vi "NIMS_NS_iir_grpdelay.vi"(5 "Function name":string, 6 "Line number":i32, 7 "Number of outputs requested":i32, 8 "error in (no error)":errorcluster, 11 "[A]":variant[](array[variant])) -> (0 "error out":errorcluster, 3 "[funct(A)]":variant[](array[variant]))   [LabVIEW 2017]
uses:
  <vilib>/imath/engines/lvmath/Functions/Error Handling/error.ctl
  <instcachedir>/0/NIMS_RunTimeType_From StrictType (excl LVString)_1019F277F0A747EDBCA0F6C52CA54500.lvgen/NIMS_RunTimeType_From StrictType (excl LVString)_1019F277F0A747EDBCA0F6C52CA54500_000.vi
  <instcachedir>/0/NIMS_Get Scalar_w Error_1987D997E87247DDAC16EA23A5E9E4FC.lvgen/NIMS_Get Scalar_w Error_1987D997E87247DDAC16EA23A5E9E4FC_000.vi
  <instcachedir>/0/NIMS_Complex To Real_BE01396FDE034E8E94CEBBA1E368668D.lvgen/NIMS_Complex To Real_BE01396FDE034E8E94CEBBA1E368668D_000.vi
  <instcachedir>/0/NIMS_Get Any Vector_w Error - Matrix_9FDB8FBE264C42EDBC8FF9BA66C3EF33.lvgen/NIMS_Get Any Vector_w Error - Matrix_9FDB8FBE264C42EDBC8FF9BA66C3EF33_001.vi
  <instcachedir>/0/NIMS_Get Scalar_w Error_1987D997E87247DDAC16EA23A5E9E4FC.lvgen/NIMS_Get Scalar_w Error_1987D997E87247DDAC16EA23A5E9E4FC_003.vi
  <instcachedir>/0/NIMS_RunTimeType_To Numeric_1CBDAFC4EFAD4045A1DE52278D16738D.lvgen/NIMS_RunTimeType_To Numeric_1CBDAFC4EFAD4045A1DE52278D16738D_000.vi
  <vilib>/addons/Digital Filter Design/NI_DigFilter_MathScript.lvlib
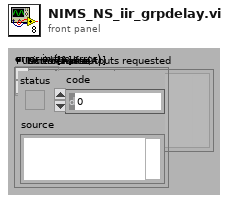
[diagram p1: front panel]
types:
  T1 = typedef "error.ctl" = enum16{"No Error", "Problem", "Input type must not be void", "Incorrect number of parameters", "Function not defined for non-numeric types", "An output variable of the user-defined function is undefined", "Function only defined for character arrays", "Function not defined for boolean, character, or single precision", "Function not defined for complex types", "Not a valid operation", "Inputs must be scalar", "Input matrices are not the same size", "Function only available on RT", "Input matrices must be nonnegative integers of the same type", "Arguments must be non-negative integers less than bitmax", "Number to complement must be less than 2^N", "Bit to get is outside range", "Bit to set is outside range", "Input must be real type ", "At least one parameter must be scalar", "Unable to display plug-in data on RT", "Function not defined for higher dimensional matrices", "Invalid attributes", "Wrong Type of Input Arguments", "Wrong Argument Option", "Invalid file identifier", "Indices must be real positive integers", "The variable is not a matrix data type.", "Number of elements must be the same for indices and values", "You cannot replace elements of a matrix with non-matrix data types.", "Cannot resize a 2D matrix with a linear index", "Unknown variable or symbol", "Indices out of range", "Empty matrix deletion can not be used with two indices", "Number of rows and columns must be the same for indices and values.", "Complex cannot be converted to Boolean", "Char cannot be converted to Boolean", "int64 cannot be converted to Boolean", "uint64 cannot be converted to Boolean", "You cannot convert a Boolean to a character.", "Incompatible input size in 3D surface function", "All rows must have the same number of columns", "Incompatible types", "Invalid matrix dimensions", "Dimension must be 1 or 2", "Base must be an integer between 2 and 36", "Invalid input", "Square matrix required", "Function 'timerstart' must be called before 'timerstop'", "Arguments must be positive real", "Step must not be zero", "Wrong number of input arguments", "Wrong number of output arguments", "Too many index arguments", "Input scalar must be >= 0", "Input scalar must be positive", "Input scalar must not be 0", "Input scalar must be in range [0,1]", "Can't use conditionally defined variable that's undefined", "Input must be a vector", "RT Exec Trace Toolkit not licensed", "Empty vector error", "All elements must be in domain [-1,1]", "All real elements of input vector must be >= 0", "All elements of input vector must be positive", "Values of input vectors are not compatible", "DAQmx not installed", "Input vector must be an increasing vector", "Dereferenced field does not exist within the struct", "A vector or matrix of structures must be indexed before it can be dereferenced", "Lenths of two input vectors are not compatible", "Invalid fieldname", "Empty matrix error", "Cannot use '.' on a type other than Struct", "Unused074", "Data type of the struct's field name is invalid", "Using . to dereference data that is not a struct", "Input struct contains invalid type ", "Size of input matrix is incompatible with input size", "Invalid format specifier", "Could not find field within struct", "Bad permutation array", "Mismatched fieldnames", "ode: User Function could not be opened", "ode: User Function signature does not meet ode requirements", "Unused085", "RunTime: MathScript could not be compiled", "Unknown function", "Only scalars and strings supported", "ode: User Function signature has incorrect number of inputs", "ode:User Function signature has incorrect number of outputs", "Range is too large", "End used without variable", "Function not available (RTE)", "Custom user error", "Arguments must be integers less than bitmax", "Shared library not found", "Header file not found", "Shared library already loaded", "Shared library not loaded", "Shared library function not found", "Shared library string return problem", "Problem calling shared library function", "Problem loading shared library from OS", "Problem parsing shared library header file", "Shared library incompatible types", "Shared library unsupported return type", "Shared library function not exported", "Shared library unsupported input type", "Problem unloading shared library from OS", "Function only available from UI", "Function specified in argument is missing", "An internal error has occurred", "Invalid object", "Invalid property", "Read-only property", "A break command has occurred", "A continue command has occurred", "A return command has occurred", "ode: times parameter invalid", "Function specified in argument has incorrect signature", "Function not found in file", "Reserved keyword cannot be defined as variable", "Reserved keyword cannot be defined as a function or script", "Arguments must be string literals", "Function not supported on this platform", "All columns must have the same number of rows", "Function ignored in RTE warning", "Cannot use : as a parameter that is not a variable", "Output can't be coerced to requested type", "Function not supported on current target", "Variable dependent on an unwired function input", "Unused132", "Unused133", "Unused134", "Unused135", "Unused136", "Unused137", "Unused138", "Unused139", "Global/Persistent must only take constants as arguments.", "Varargin must be last input in the function definition.", "Varargout must be last output in the function definition.", "Invalid output type. Cannot output a cell array of any type other than string.", "Invalid output type. Type is a dynamic struct.", "Invalid output type. Type is a struct that has a field whose type is not known until run-time", "Invalid output type. Type is a struct that has a field which is a plot object.", "MathScript parser DLL missing", "MathScript requires LabVIEW Full", "MathScript license is invalid or missing", "Varargout not supported except in assignments."}
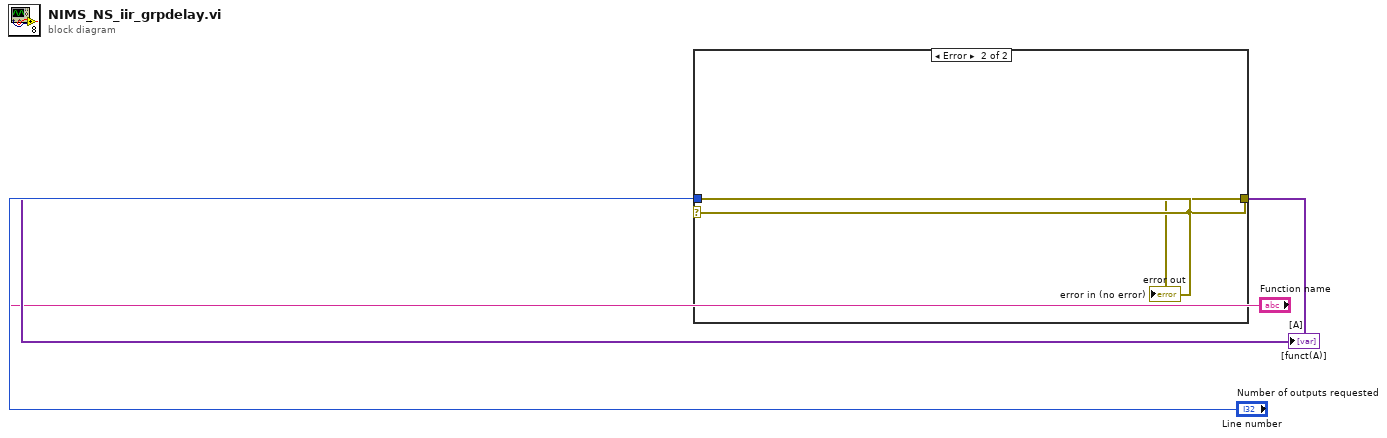
[diagram p0: block diagram]
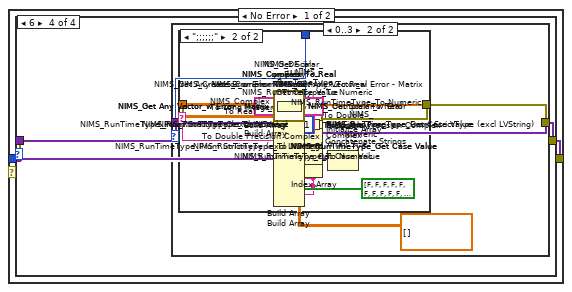
[diagram p2: hidden frame]
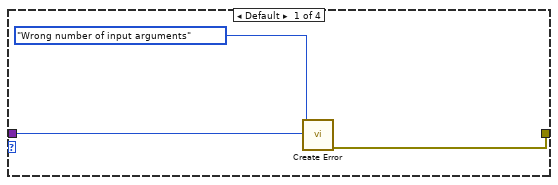
[diagram p3: hidden frame]
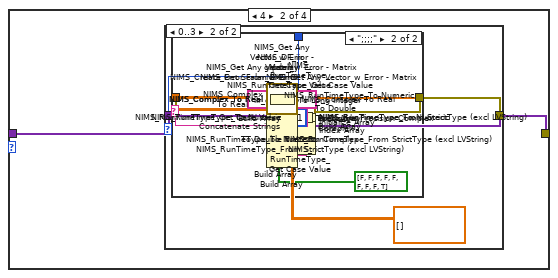
[diagram p4: hidden frame]
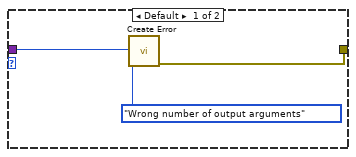
[diagram p5: hidden frame]
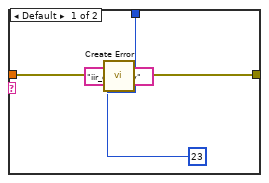
[diagram p6: hidden frame]
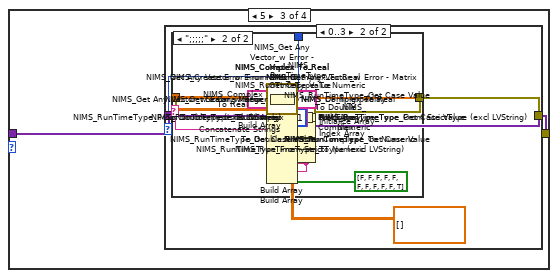
[diagram p7: hidden frame]
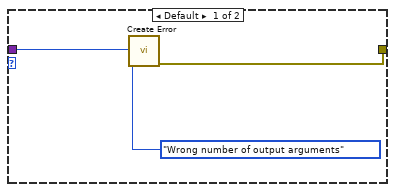
[diagram p8: hidden frame]
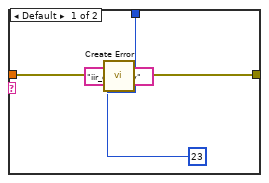
[diagram p9: hidden frame]
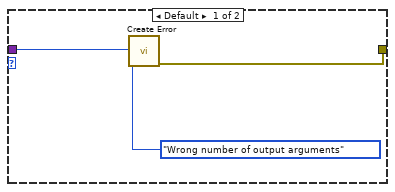
[diagram p10: hidden frame]
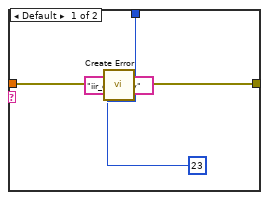
[diagram p11: hidden frame]
diagram:
  n1 = case shown="Error" "error in (no error)" {
    selector: "error in (no error)" -> [_ w312]
    tunnel: [w15 _] -> w4
    tunnel: [w14 w312] -> w3
    tunnel: "error in (no error)" -> [w13 _]
    tunnel: "Number of outputs requested" -> [w12 _]
    tunnel: "[A]" -> [w11 _]
    tunnel: "Function name" -> [w10 _]
    tunnel: "Line number" -> [w9 _]
    frame No Error {
      n2 = Array Size(array=w11) -> (size(s)=w8:i32)
      n3 = case shown="6" w8 {
        tunnel: [_ w27 w115 w212] -> w15
        tunnel: w10 -> [w19 w24 w112 w209]
        tunnel: w9 -> [w20 w25 w113 w210]
        tunnel: w13 -> [w17 w23 w111 w208]
        tunnel: [w16 w22 w110 w207] -> w14
        tunnel: w12 -> [_ w21 w109 w206]
        tunnel: w11 -> [_ w26 w114 w211]
        frame Default {
          n4 = call <vilib>:"Create Error.vi"("Function name"=w19, "error in (no error)"=w17, "Error Enum"=error."Wrong number of input arguments", "Line number"=w20) -> ("error out"=w16:errorcluster)  [unwired: 6 in, 1 out]
        }
        frame 4 {
          n5 = case shown="0..3" w21 {
            tunnel: [_ w33] -> w27
            tunnel: w24 -> [w31 _]
            tunnel: w25 -> [w32 w69]
            tunnel: w23 -> [w29 w67]
            tunnel: [w28 w50] -> w22
            tunnel: w26 -> [_ w70]
            frame Default {
              n6 = call <vilib>:"Create Error.vi"("Function name"=w31, "error in (no error)"=w29, "Error Enum"=error."Wrong number of output arguments", "Line number"=w32) -> ("error out"=w28:errorcluster)  [unwired: 6 in, 1 out]
            }
            frame 0..3 {
              w40 = 1
              n7 = Index Array(array=w70) -> (element #1=w66:variant, element #2=w62:variant, element #3=w58:variant, element #4=w54:variant)  [unwired: 4 in]
              n8 = call <vilib>:"NIMS_RunTimeType_Get Case Value.vi"("Data In"=w54) -> ("Case Value"=w51:string)  [unwired: 9 in, 1 out]
              n9 = call-generic <vilib>:"NIMS_RunTimeType_To Numeric.vi"("DataType"=cdb[][] [], "Variant"=w54) -> ("data"=w52:cdb[][])  [unwired: 1 in]
              n10 = call <vilib>:"NIMS_RunTimeType_Get Case Value.vi"("Data In"=w58) -> ("Case Value"=w55:string)  [unwired: 9 in, 1 out]
              n11 = call-generic <vilib>:"NIMS_RunTimeType_To Numeric.vi"("DataType"=cdb[][] [], "Variant"=w58) -> ("data"=w56:cdb[][])  [unwired: 1 in]
              n12 = call <vilib>:"NIMS_RunTimeType_Get Case Value.vi"("Data In"=w62) -> ("Case Value"=w59:string)  [unwired: 9 in, 1 out]
              n13 = call-generic <vilib>:"NIMS_RunTimeType_To Numeric.vi"("DataType"=cdb[][] [], "Variant"=w62) -> ("data"=w60:cdb[][])  [unwired: 1 in]
              n14 = call <vilib>:"NIMS_RunTimeType_Get Case Value.vi"("Data In"=w66) -> ("Case Value"=w63:string)  [unwired: 9 in, 1 out]
              n15 = call-generic <vilib>:"NIMS_RunTimeType_To Numeric.vi"("DataType"=cdb[][] [], "Variant"=w66) -> ("data"=w64:cdb[][])  [unwired: 1 in]
              n16 = Concatenate Strings(w63, w59, w55, w51) -> (w68:string)
              n17 = case shown="\";;;;\"" w68 {
                tunnel: w67 -> [w72 w83]
                tunnel: [_ w78] -> w49
                tunnel: [_ w77] -> w45
                tunnel: [_ w76] -> w41
                tunnel: [w71 w79] -> w50
                tunnel: w64 -> [_ w107]
                tunnel: w60 -> [_ w103]
                tunnel: w56 -> [_ w100]
                tunnel: w52 -> [_ w97]
                tunnel: w69 -> [w75 w86]
                frame Default {
                  n18 = call <vilib>:"Create Error.vi"("Function name"="iir_grpdelay", "error in (no error)"=w72, "Error Enum"=23, "Line number"=w75) -> ("error out"=w71:errorcluster)  [unwired: 6 in, 1 out]
                }
                frame ";;;;" {
                  w81 = "iir_grpdelay"
                  n19 = call-generic <vilib>:"NIMS_Complex To Real.vi"("A"=w97) -> ("Error Enum"=w89:T1, "Real(A)"=w96:dbl[][])  [unwired: 8 in, 1 out]
                  n20 = call-generic <vilib>:"NIMS_Get Any Vector_w Error - Matrix.vi"("A"=w96) -> ("Error Enum"=w88:T1, "Vector"=w98:dbl[])  [unwired: 8 in, 1 out]
                  n21 = call-generic <vilib>:"NIMS_Complex To Real.vi"("A"=w100) -> ("Error Enum"=w91:T1, "Real(A)"=w99:dbl[][])  [unwired: 8 in, 1 out]
                  n22 = call-generic <vilib>:"NIMS_Get Any Vector_w Error - Matrix.vi"("A"=w99) -> ("Error Enum"=w90:T1, "Vector"=w101:dbl[])  [unwired: 8 in, 1 out]
                  n23 = call-generic <vilib>:"NIMS_Complex To Real.vi"("A"=w103) -> ("Error Enum"=w93:T1, "Real(A)"=w102:dbl[][])  [unwired: 8 in, 1 out]
                  n24 = call-generic <vilib>:"NIMS_Get Any Vector_w Error - Matrix.vi"("A"=w102) -> ("Error Enum"=w92:T1, "Vector"=w104:dbl[])  [unwired: 8 in, 1 out]
                  n25 = call-generic <vilib>:"NIMS_Complex To Real.vi"("A"=w107) -> ("Error Enum"=w95:T1, "Real(A)"=w106:dbl[][])  [unwired: 8 in, 1 out]
                  n26 = To Long Integer(number=w106) -> (32bit integer=w105:i32[][])
                  n27 = call-generic <vilib>:"NIMS_Get Scalar_w Error.vi"("A"=w105) -> ("Error Enum"=w94:T1, "Scalar"=w108:i32)  [unwired: 8 in, 1 out]
                  n28 = call <vilib>:"NIMS_DF_iir_grpdelay.vi"("grp"=w98, "e"=w101, "f"=w104, "n"=w108) -> ("error"=w87:i32, "offset"=w76:dbl, "a"=w77:dbl[], "b"=w78:dbl[])  [unwired: 4 in]
                  n29 = Build Array(w81, w81, w81, w81, w81, w81, w81, w81, "iir_grpdelay") -> (w84:string[])
                  n30 = Build Array(w95, w94, w93, w92, w91, w90, w89, w88, w87) -> (w85:i32[])
                  n31 = call <vilib>:"NIMS_Create Error From Enums.vi"("Error Code"=bool[] [FALSE, FALSE, FALSE, FALSE, FALSE, FALSE, FALSE, FALSE, TRUE], "error in (no error)"=w83, "Line no"=w86, "Error Enums"=w85, "Function names"=w84) -> ("error out"=w79:errorcluster)  [unwired: 6 in]
                }
              }
              n32 = Initialize Array(w41, w40, w40) -> (w39:dbl[][])
              n33 = To Double Precision Complex(1:w39) -> (0:w38:cdb[][])
              n34 = call-generic <vilib>:"NIMS_RunTimeType_From StrictType (excl LVString).vi"("Plug-In Name"="", "Data In"=w38) -> ("Data Out"=w34:variant)  [unwired: 2 in]
              n35 = Build Array(w45) -> (w44:dbl[][])
              n36 = To Double Precision Complex(1:w44) -> (0:w43:cdb[][])
              n37 = call-generic <vilib>:"NIMS_RunTimeType_From StrictType (excl LVString).vi"("Plug-In Name"="", "Data In"=w43) -> ("Data Out"=w35:variant)  [unwired: 2 in]
              n38 = Build Array(w49) -> (w48:dbl[][])
              n39 = To Double Precision Complex(1:w48) -> (0:w47:cdb[][])
              n40 = call-generic <vilib>:"NIMS_RunTimeType_From StrictType (excl LVString).vi"("Plug-In Name"="", "Data In"=w47) -> ("Data Out"=w36:variant)  [unwired: 2 in]
              n41 = Build Array(w36, w35, w34) -> (w33:variant[])
            }
          }
        }
        frame 5 {
          n42 = case shown="0..3" w109 {
            tunnel: [_ w121] -> w115
            tunnel: w112 -> [w119 _]
            tunnel: w113 -> [w120 w161]
            tunnel: w111 -> [w117 w159]
            tunnel: [w116 w138] -> w110
            tunnel: w114 -> [_ w162]
            frame Default {
              n43 = call <vilib>:"Create Error.vi"("Function name"=w119, "error in (no error)"=w117, "Error Enum"=error."Wrong number of output arguments", "Line number"=w120) -> ("error out"=w116:errorcluster)  [unwired: 6 in, 1 out]
            }
            frame 0..3 {
              w128 = 1
              n44 = Index Array(array=w162) -> (element #1=w158:variant, element #2=w154:variant, element #3=w150:variant, element #4=w146:variant, element #5=w142:variant)  [unwired: 5 in]
              n45 = call <vilib>:"NIMS_RunTimeType_Get Case Value.vi"("Data In"=w142) -> ("Case Value"=w139:string)  [unwired: 9 in, 1 out]
              n46 = call-generic <vilib>:"NIMS_RunTimeType_To Numeric.vi"("DataType"=cdb[][] [], "Variant"=w142) -> ("data"=w140:cdb[][])  [unwired: 1 in]
              n47 = call <vilib>:"NIMS_RunTimeType_Get Case Value.vi"("Data In"=w146) -> ("Case Value"=w143:string)  [unwired: 9 in, 1 out]
              n48 = call-generic <vilib>:"NIMS_RunTimeType_To Numeric.vi"("DataType"=cdb[][] [], "Variant"=w146) -> ("data"=w144:cdb[][])  [unwired: 1 in]
              n49 = call <vilib>:"NIMS_RunTimeType_Get Case Value.vi"("Data In"=w150) -> ("Case Value"=w147:string)  [unwired: 9 in, 1 out]
              n50 = call-generic <vilib>:"NIMS_RunTimeType_To Numeric.vi"("DataType"=cdb[][] [], "Variant"=w150) -> ("data"=w148:cdb[][])  [unwired: 1 in]
              n51 = call <vilib>:"NIMS_RunTimeType_Get Case Value.vi"("Data In"=w154) -> ("Case Value"=w151:string)  [unwired: 9 in, 1 out]
              n52 = call-generic <vilib>:"NIMS_RunTimeType_To Numeric.vi"("DataType"=cdb[][] [], "Variant"=w154) -> ("data"=w152:cdb[][])  [unwired: 1 in]
              n53 = call <vilib>:"NIMS_RunTimeType_Get Case Value.vi"("Data In"=w158) -> ("Case Value"=w155:string)  [unwired: 9 in, 1 out]
              n54 = call-generic <vilib>:"NIMS_RunTimeType_To Numeric.vi"("DataType"=cdb[][] [], "Variant"=w158) -> ("data"=w156:cdb[][])  [unwired: 1 in]
              n55 = Concatenate Strings(w155, w151, w147, w143, w139) -> (w160:string)
              n56 = case shown="\";;;;;\"" w160 {
                tunnel: w159 -> [w164 w175]
                tunnel: [_ w170] -> w137
                tunnel: [_ w169] -> w133
                tunnel: [_ w168] -> w129
                tunnel: [w163 w171] -> w138
                tunnel: w156 -> [_ w204]
                tunnel: w152 -> [_ w200]
                tunnel: w148 -> [_ w197]
                tunnel: w144 -> [_ w194]
                tunnel: w140 -> [_ w191]
                tunnel: w161 -> [w167 w178]
                frame Default {
                  n57 = call <vilib>:"Create Error.vi"("Function name"="iir_grpdelay", "error in (no error)"=w164, "Error Enum"=23, "Line number"=w167) -> ("error out"=w163:errorcluster)  [unwired: 6 in, 1 out]
                }
                frame ";;;;;" {
                  w173 = "iir_grpdelay"
                  n58 = call-generic <vilib>:"NIMS_Complex To Real.vi"("A"=w191) -> ("Error Enum"=w181:T1, "Real(A)"=w190:dbl[][])  [unwired: 8 in, 1 out]
                  n59 = call-generic <vilib>:"NIMS_Get Any Vector_w Error - Matrix.vi"("A"=w190) -> ("Error Enum"=w180:T1, "Vector"=w192:dbl[])  [unwired: 8 in, 1 out]
                  n60 = call-generic <vilib>:"NIMS_Complex To Real.vi"("A"=w194) -> ("Error Enum"=w183:T1, "Real(A)"=w193:dbl[][])  [unwired: 8 in, 1 out]
                  n61 = call-generic <vilib>:"NIMS_Get Any Vector_w Error - Matrix.vi"("A"=w193) -> ("Error Enum"=w182:T1, "Vector"=w195:dbl[])  [unwired: 8 in, 1 out]
                  n62 = call-generic <vilib>:"NIMS_Complex To Real.vi"("A"=w197) -> ("Error Enum"=w185:T1, "Real(A)"=w196:dbl[][])  [unwired: 8 in, 1 out]
                  n63 = call-generic <vilib>:"NIMS_Get Any Vector_w Error - Matrix.vi"("A"=w196) -> ("Error Enum"=w184:T1, "Vector"=w198:dbl[])  [unwired: 8 in, 1 out]
                  n64 = call-generic <vilib>:"NIMS_Complex To Real.vi"("A"=w200) -> ("Error Enum"=w187:T1, "Real(A)"=w199:dbl[][])  [unwired: 8 in, 1 out]
                  n65 = call-generic <vilib>:"NIMS_Get Any Vector_w Error - Matrix.vi"("A"=w199) -> ("Error Enum"=w186:T1, "Vector"=w201:dbl[])  [unwired: 8 in, 1 out]
                  n66 = call-generic <vilib>:"NIMS_Complex To Real.vi"("A"=w204) -> ("Error Enum"=w189:T1, "Real(A)"=w203:dbl[][])  [unwired: 8 in, 1 out]
                  n67 = To Long Integer(number=w203) -> (32bit integer=w202:i32[][])
                  n68 = call-generic <vilib>:"NIMS_Get Scalar_w Error.vi"("A"=w202) -> ("Error Enum"=w188:T1, "Scalar"=w205:i32)  [unwired: 8 in, 1 out]
                  n69 = call <vilib>:"NIMS_DF_iir_grpdelay.vi"("w"=w192, "grp"=w195, "e"=w198, "f"=w201, "n"=w205) -> ("error"=w179:i32, "offset"=w168:dbl, "a"=w169:dbl[], "b"=w170:dbl[])  [unwired: 3 in]
                  n70 = Build Array(w173, w173, w173, w173, w173, w173, w173, w173, w173, w173, "iir_grpdelay") -> (w176:string[])
                  n71 = Build Array(w189, w188, w187, w186, w185, w184, w183, w182, w181, w180, w179) -> (w177:i32[])
                  n72 = call <vilib>:"NIMS_Create Error From Enums.vi"("Error Code"=bool[] [FALSE, FALSE, FALSE, FALSE, FALSE, FALSE, FALSE, FALSE, FALSE, FALSE, TRUE], "error in (no error)"=w175, "Line no"=w178, "Error Enums"=w177, "Function names"=w176) -> ("error out"=w171:errorcluster)  [unwired: 6 in]
                }
              }
              n73 = Initialize Array(w129, w128, w128) -> (w127:dbl[][])
              n74 = To Double Precision Complex(1:w127) -> (0:w126:cdb[][])
              n75 = call-generic <vilib>:"NIMS_RunTimeType_From StrictType (excl LVString).vi"("Plug-In Name"="", "Data In"=w126) -> ("Data Out"=w122:variant)  [unwired: 2 in]
              n76 = Build Array(w133) -> (w132:dbl[][])
              n77 = To Double Precision Complex(1:w132) -> (0:w131:cdb[][])
              n78 = call-generic <vilib>:"NIMS_RunTimeType_From StrictType (excl LVString).vi"("Plug-In Name"="", "Data In"=w131) -> ("Data Out"=w123:variant)  [unwired: 2 in]
              n79 = Build Array(w137) -> (w136:dbl[][])
              n80 = To Double Precision Complex(1:w136) -> (0:w135:cdb[][])
              n81 = call-generic <vilib>:"NIMS_RunTimeType_From StrictType (excl LVString).vi"("Plug-In Name"="", "Data In"=w135) -> ("Data Out"=w124:variant)  [unwired: 2 in]
              n82 = Build Array(w124, w123, w122) -> (w121:variant[])
            }
          }
        }
        frame 6 {
          n83 = case shown="0..3" w206 {
            tunnel: [_ w218] -> w212
            tunnel: w209 -> [w216 _]
            tunnel: w210 -> [w217 w262]
            tunnel: w208 -> [w214 w260]
            tunnel: [w213 w235] -> w207
            tunnel: w211 -> [_ w263]
            frame Default {
              n84 = call <vilib>:"Create Error.vi"("Function name"=w216, "error in (no error)"=w214, "Error Enum"=error."Wrong number of output arguments", "Line number"=w217) -> ("error out"=w213:errorcluster)  [unwired: 6 in, 1 out]
            }
            frame 0..3 {
              w225 = 1
              n85 = Index Array(array=w263) -> (element #1=w259:variant, element #2=w255:variant, element #3=w251:variant, element #4=w247:variant, element #5=w243:variant, element #6=w239:variant)  [unwired: 6 in]
              n86 = call <vilib>:"NIMS_RunTimeType_Get Case Value.vi"("Data In"=w239) -> ("Case Value"=w236:string)  [unwired: 9 in, 1 out]
              n87 = call-generic <vilib>:"NIMS_RunTimeType_To Numeric.vi"("DataType"=cdb[][] [], "Variant"=w239) -> ("data"=w237:cdb[][])  [unwired: 1 in]
              n88 = call <vilib>:"NIMS_RunTimeType_Get Case Value.vi"("Data In"=w243) -> ("Case Value"=w240:string)  [unwired: 9 in, 1 out]
              n89 = call-generic <vilib>:"NIMS_RunTimeType_To Numeric.vi"("DataType"=cdb[][] [], "Variant"=w243) -> ("data"=w241:cdb[][])  [unwired: 1 in]
              n90 = call <vilib>:"NIMS_RunTimeType_Get Case Value.vi"("Data In"=w247) -> ("Case Value"=w244:string)  [unwired: 9 in, 1 out]
              n91 = call-generic <vilib>:"NIMS_RunTimeType_To Numeric.vi"("DataType"=cdb[][] [], "Variant"=w247) -> ("data"=w245:cdb[][])  [unwired: 1 in]
              n92 = call <vilib>:"NIMS_RunTimeType_Get Case Value.vi"("Data In"=w251) -> ("Case Value"=w248:string)  [unwired: 9 in, 1 out]
              n93 = call-generic <vilib>:"NIMS_RunTimeType_To Numeric.vi"("DataType"=cdb[][] [], "Variant"=w251) -> ("data"=w249:cdb[][])  [unwired: 1 in]
              n94 = call <vilib>:"NIMS_RunTimeType_Get Case Value.vi"("Data In"=w255) -> ("Case Value"=w252:string)  [unwired: 9 in, 1 out]
              n95 = call-generic <vilib>:"NIMS_RunTimeType_To Numeric.vi"("DataType"=cdb[][] [], "Variant"=w255) -> ("data"=w253:cdb[][])  [unwired: 1 in]
              n96 = call <vilib>:"NIMS_RunTimeType_Get Case Value.vi"("Data In"=w259) -> ("Case Value"=w256:string)  [unwired: 9 in, 1 out]
              n97 = call-generic <vilib>:"NIMS_RunTimeType_To Numeric.vi"("DataType"=cdb[][] [], "Variant"=w259) -> ("data"=w257:cdb[][])  [unwired: 1 in]
              n98 = Concatenate Strings(w256, w252, w248, w244, w240, w236) -> (w261:string)
              n99 = case shown="\";;;;;;\"" w261 {
                tunnel: w260 -> [w265 w276]
                tunnel: [_ w271] -> w234
                tunnel: [_ w270] -> w230
                tunnel: [_ w269] -> w226
                tunnel: [w264 w272] -> w235
                tunnel: w257 -> [_ w310]
                tunnel: w253 -> [_ w306]
                tunnel: w249 -> [_ w303]
                tunnel: w245 -> [_ w300]
                tunnel: w241 -> [_ w297]
                tunnel: w237 -> [_ w294]
                tunnel: w262 -> [w268 w279]
                frame Default {
                  n100 = call <vilib>:"Create Error.vi"("Function name"="iir_grpdelay", "error in (no error)"=w265, "Error Enum"=23, "Line number"=w268) -> ("error out"=w264:errorcluster)  [unwired: 6 in, 1 out]
                }
                frame ";;;;;;" {
                  w274 = "iir_grpdelay"
                  n101 = call-generic <vilib>:"NIMS_Complex To Real.vi"("A"=w294) -> ("Error Enum"=w282:T1, "Real(A)"=w293:dbl[][])  [unwired: 8 in, 1 out]
                  n102 = call-generic <vilib>:"NIMS_Get Scalar_w Error.vi"("A"=w293) -> ("Error Enum"=w281:T1, "Scalar"=w295:dbl)  [unwired: 8 in, 1 out]
                  n103 = call-generic <vilib>:"NIMS_Complex To Real.vi"("A"=w297) -> ("Error Enum"=w284:T1, "Real(A)"=w296:dbl[][])  [unwired: 8 in, 1 out]
                  n104 = call-generic <vilib>:"NIMS_Get Any Vector_w Error - Matrix.vi"("A"=w296) -> ("Error Enum"=w283:T1, "Vector"=w298:dbl[])  [unwired: 8 in, 1 out]
                  n105 = call-generic <vilib>:"NIMS_Complex To Real.vi"("A"=w300) -> ("Error Enum"=w286:T1, "Real(A)"=w299:dbl[][])  [unwired: 8 in, 1 out]
                  n106 = call-generic <vilib>:"NIMS_Get Any Vector_w Error - Matrix.vi"("A"=w299) -> ("Error Enum"=w285:T1, "Vector"=w301:dbl[])  [unwired: 8 in, 1 out]
                  n107 = call-generic <vilib>:"NIMS_Complex To Real.vi"("A"=w303) -> ("Error Enum"=w288:T1, "Real(A)"=w302:dbl[][])  [unwired: 8 in, 1 out]
                  n108 = call-generic <vilib>:"NIMS_Get Any Vector_w Error - Matrix.vi"("A"=w302) -> ("Error Enum"=w287:T1, "Vector"=w304:dbl[])  [unwired: 8 in, 1 out]
                  n109 = call-generic <vilib>:"NIMS_Complex To Real.vi"("A"=w306) -> ("Error Enum"=w290:T1, "Real(A)"=w305:dbl[][])  [unwired: 8 in, 1 out]
                  n110 = call-generic <vilib>:"NIMS_Get Any Vector_w Error - Matrix.vi"("A"=w305) -> ("Error Enum"=w289:T1, "Vector"=w307:dbl[])  [unwired: 8 in, 1 out]
                  n111 = call-generic <vilib>:"NIMS_Complex To Real.vi"("A"=w310) -> ("Error Enum"=w292:T1, "Real(A)"=w309:dbl[][])  [unwired: 8 in, 1 out]
                  n112 = To Long Integer(number=w309) -> (32bit integer=w308:i32[][])
                  n113 = call-generic <vilib>:"NIMS_Get Scalar_w Error.vi"("A"=w308) -> ("Error Enum"=w291:T1, "Scalar"=w311:i32)  [unwired: 8 in, 1 out]
                  n114 = call <vilib>:"NIMS_DF_iir_grpdelay.vi"("r"=w295, "w"=w298, "grp"=w301, "e"=w304, "f"=w307, "n"=w311) -> ("error"=w280:i32, "offset"=w269:dbl, "a"=w270:dbl[], "b"=w271:dbl[])  [unwired: 2 in]
                  n115 = Build Array(w274, w274, w274, w274, w274, w274, w274, w274, w274, w274, w274, w274, "iir_grpdelay") -> (w277:string[])
                  n116 = Build Array(w292, w291, w290, w289, w288, w287, w286, w285, w284, w283, w282, w281, w280) -> (w278:i32[])
                  n117 = call <vilib>:"NIMS_Create Error From Enums.vi"("Error Code"=bool[] [FALSE, FALSE, FALSE, FALSE, FALSE, FALSE, FALSE, FALSE, FALSE, FALSE, FALSE, FALSE, TRUE], "error in (no error)"=w276, "Line no"=w279, "Error Enums"=w278, "Function names"=w277) -> ("error out"=w272:errorcluster)  [unwired: 6 in]
                }
              }
              n118 = Initialize Array(w226, w225, w225) -> (w224:dbl[][])
              n119 = To Double Precision Complex(1:w224) -> (0:w223:cdb[][])
              n120 = call-generic <vilib>:"NIMS_RunTimeType_From StrictType (excl LVString).vi"("Plug-In Name"="", "Data In"=w223) -> ("Data Out"=w219:variant)  [unwired: 2 in]
              n121 = Build Array(w230) -> (w229:dbl[][])
              n122 = To Double Precision Complex(1:w229) -> (0:w228:cdb[][])
              n123 = call-generic <vilib>:"NIMS_RunTimeType_From StrictType (excl LVString).vi"("Plug-In Name"="", "Data In"=w228) -> ("Data Out"=w220:variant)  [unwired: 2 in]
              n124 = Build Array(w234) -> (w233:dbl[][])
              n125 = To Double Precision Complex(1:w233) -> (0:w232:cdb[][])
              n126 = call-generic <vilib>:"NIMS_RunTimeType_From StrictType (excl LVString).vi"("Plug-In Name"="", "Data In"=w232) -> ("Data Out"=w221:variant)  [unwired: 2 in]
              n127 = Build Array(w221, w220, w219) -> (w218:variant[])
            }
          }
        }
      }
    }
    frame Error {
    }
  }
  "error out" <- w3
  "[funct(A)]" <- w4
